vi "SimpleCalculatorInvokeNode.vi"() -> ()   [LabVIEW 2019]
panel:
  in  "stop":bool
  in  "Div":bool
  in  "Mul":bool
  in  "Sub":bool
  in  "Add":bool
  out "c":dbl
  in  "b":dbl
  in  "a":dbl
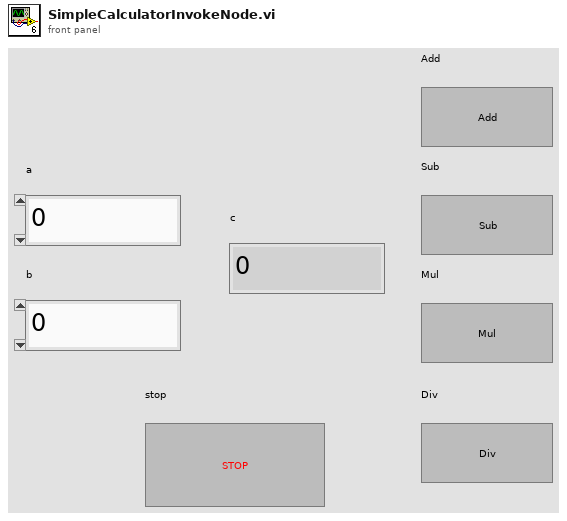
[diagram p1: front panel]
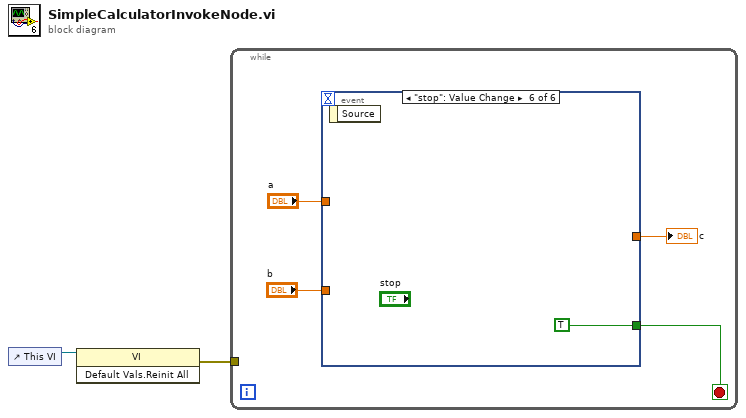
[diagram p0: block diagram]
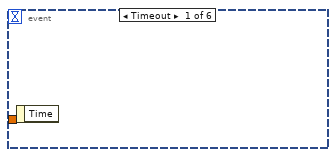
[diagram p2: hidden frame]
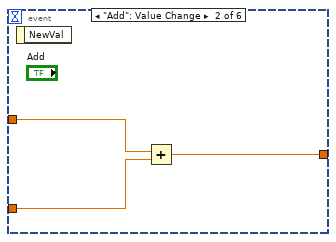
[diagram p3: hidden frame]
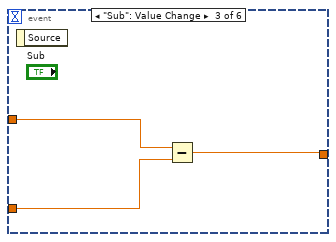
[diagram p4: hidden frame]
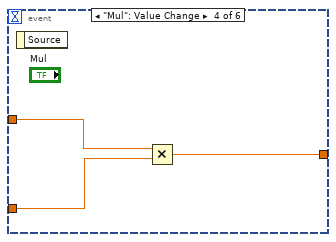
[diagram p5: hidden frame]
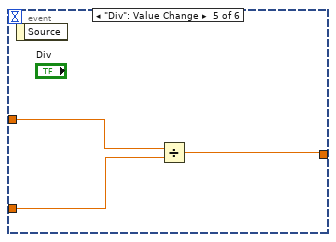
[diagram p6: hidden frame]
diagram:
  n1 = control-ref of="This VI"() -> (w2:refnum<vi>)
  n2 = invoke class="VI" method="Default Vals.Reinit All"(reference=w2) -> (error out=w1:errorcluster)  [unwired: 2 in, 2 out]
  n3 = while {
    tunnel: w1 -> [_]
    stop <- w3 stop-if-true
    n4 = event shown="[5] \"stop\": Value Change" {
      selector: _ -> [_ _ _ _ _ _]
      dyn-events: _ -> [_ _ _ _ _ _]
      timeout: _ -> [_ _ _ _ _ _]
      tunnel: "a" -> [_ w9 w12 w15 w18 _]
      tunnel: "b" -> [_ w8 w11 w14 w17 _]
      tunnel: [_ w7 w10 w13 w16 _] -> w4
      tunnel: [_ _ _ _ _ TRUE] -> w3
      event Timeout {
        n5 = event-data() -> ()  [unwired: 1 in, 1 out]
      }
      event "Add": Value Change {
        n6 = event-data() -> ()  [unwired: 1 in, 1 out]
        n7 = Add(x=w9, y=w8) -> (x+y=w7:dbl)
      }
      event "Sub": Value Change {
        n8 = event-data() -> ()  [unwired: 1 in, 1 out]
        n9 = Subtract(x=w12, y=w11) -> (x-y=w10:dbl)
      }
      event "Mul": Value Change {
        n10 = event-data() -> ()  [unwired: 1 in, 1 out]
        n11 = Multiply(x=w15, y=w14) -> (x*y=w13:dbl)
      }
      event "Div": Value Change {
        n12 = event-data() -> ()  [unwired: 1 in, 1 out]
        n13 = Divide(x=w18, y=w17) -> (x/y=w16:dbl)
      }
      event "stop": Value Change {
        n14 = event-data() -> ()  [unwired: 1 in, 1 out]
      }
    }
    "c" <- w4
  }
